vi "Class Data Type.vi"(8 "error in (no error)":errorcluster, 11 "GroupAbstract in":refnum<class "GroupAbstract.lvclass">) -> (0 "error out":errorcluster, 2 "Class Data Type":T1, 3 "GroupAbstract out":refnum<class "GroupAbstract.lvclass">)   [LabVIEW 2020, in "Vecto.lvlib" / "GroupAbstract.lvclass"]
uses:
  GroupAbstract.lvclass
  Group Data Type.ctl
  GroupAbstract.lvclass/GroupAbstract.ctl
  VectoConfig/VectoConfig.lvlib
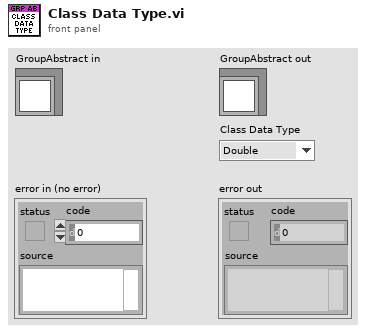
[diagram p1: front panel]
types:
  T1 = typedef "VectoConfig.lvlib/Group Data Type.ctl" = enum16{"Double", "String"}
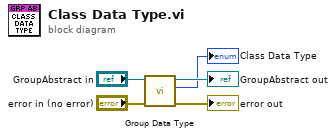
[diagram p0: block diagram]
diagram:
  n1 = call-dynamic "Group Data Type.vi"("error in (no error)"="error in (no error)", "GroupAbstract in"="GroupAbstract in") -> ("error out"=→"error out":errorcluster, "Group Data Type"=→"Class Data Type":T1, "GroupAbstract out"=→"GroupAbstract out":refnum<class "GroupAbstract.lvclass">)  [unwired: 7 in]
